vi "Read Sprites.vi"(8 "error in (no error)":errorcluster, 11 "Game in":refnum<class "Game.lvclass">) -> (0 "error out":errorcluster, 2 "Sprites":T1, 3 "Game out":refnum<class "Game.lvclass">)   [LabVIEW 2019, in "RT_Game.lvlib" / "Game.lvclass"]
uses:
  Game.lvclass
  SpritesCluster.ctl
  RT_Sprite/RT_Sprite.lvclass
  Game.lvclass/Game.ctl
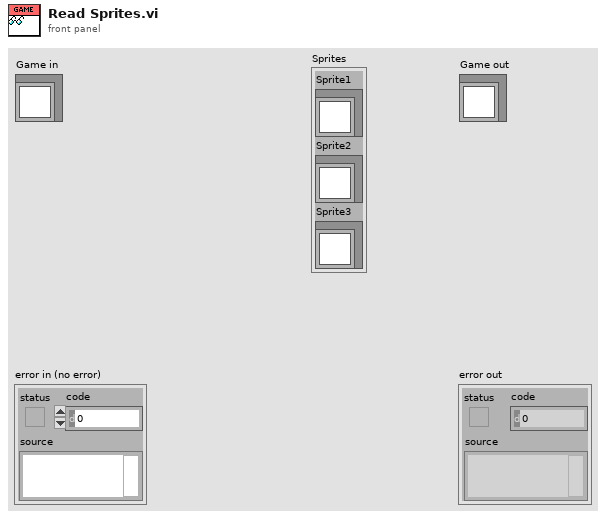
[diagram p1: front panel]
types:
  T1 = typedef "RT_Game.lvlib/Game.lvclass/SpritesCluster.ctl" = cluster{"Sprite1":refnum<class "RT_Sprite.lvclass">, "Sprite2":refnum<class "RT_Sprite.lvclass">, "Sprite3":refnum<class "RT_Sprite.lvclass">}
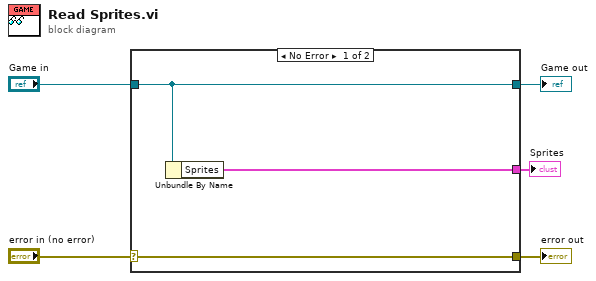
[diagram p0: block diagram]
diagram:
  n1 = case shown="No Error" "error in (no error)" {
    selector: "error in (no error)" -> [w8 w9]
    tunnel: [w8 w9] -> w4
    tunnel: [w7 w10] -> w2
    tunnel: "Game in" -> [w7 w10]
    tunnel: [w6 _] -> w1
    frame No Error {
      n2 = Unbundle By Name(w7) -> ("Sprites"=w6:T1)
    }
    frame Error {
    }
  }
  "error out" <- w4
  "Game out" <- w2
  "Sprites" <- w1
